vi "Set XY Scale Properties on Variant.vi"(8 "error in (no error)":errorcluster, 10 "Scale Properties":T1 {"X.Format" items=["Decimal", "Scientific", "Engineering", "Binary", "Octal", "Hexadecimal", "Relative Time", "Time and Date", "SI", "Automatic"]; "Y.Precision:" items=["0", "1", "2", "3", "4", "5", "6", "7"]; "Y.Format" items=["Decimal", "Scientific", "Engineering", "Binary", "Octal", "Hexadecimal", "Relative Time", "Time and Date", "SI", "Automatic"]; "X.Precision" items=["0", "1", "2", "3", "4", "5", "6", "7"]}, 11 "variant in":variant) -> (0 "error out":errorcluster, 3 "variant out":variant)   [LabVIEW 2020, in "Workspace MultiY Graph.lvlib"]
uses:
  Workspace MultiY Graph.lvlib
  XY Scale Properties.ctl
  XY Scale Precision.ctl
  XY Scale Format.ctl
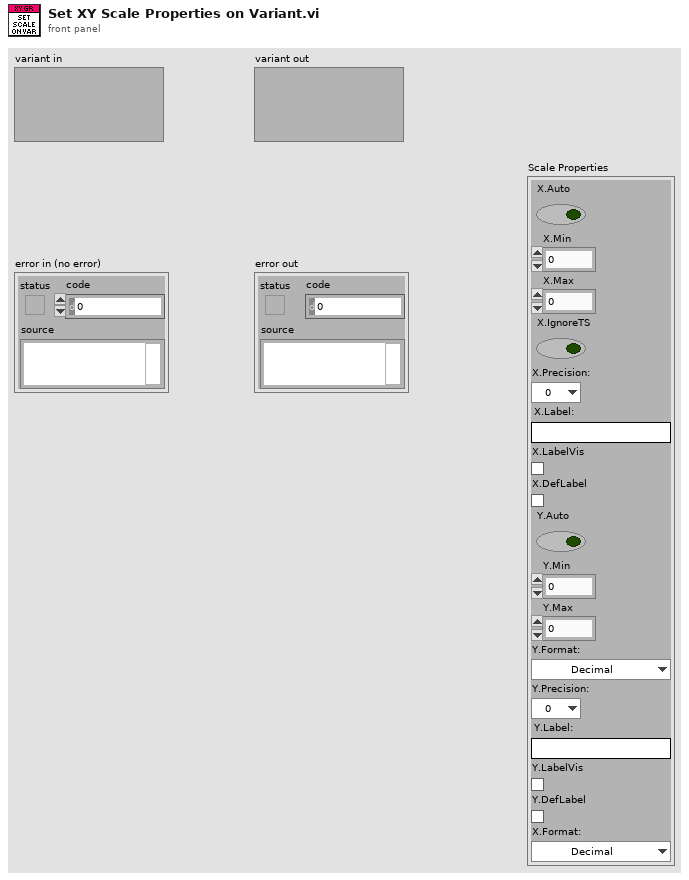
[diagram p1: front panel]
types:
  T1 = typedef "Workspace MultiY Graph.lvlib/XY Scale Properties.ctl" = cluster{"X.Auto":bool, "X.Min":dbl, "X.Max":dbl, "X.IgnoreTS":bool, "X.Precision":T2, "X.Label:":string, "X.LabelVis":bool, "X.DefLabel":bool, "Y.Auto":bool, "Y.Min":dbl, "Y.Max":dbl, "Y.Format":T3, "Y.Precision:":T2, "Y.Label:":string, "Y.LabelVis":bool, "Y.DefLabel":bool, "X.Format":T3}
  T2 = typedef "Workspace MultiY Graph.lvlib/XY Scale Precision.ctl" = u8
  T3 = typedef "Workspace MultiY Graph.lvlib/XY Scale Format.ctl" = u8
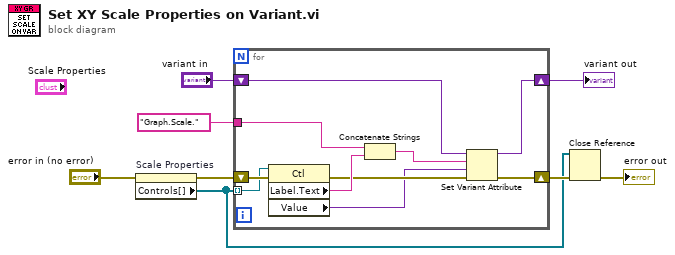
[diagram p0: block diagram]
diagram:
  n1 = property on="Scale Properties" class="Clust (strict)"(error in="error in (no error)") -> (error out=w8:errorcluster, "Controls[]"=w4:refnum<vi>[])  [unwired: 1 in, 1 out]
  n2 = for {
    tunnel: w4 -> [w17] mode=indexing
    tunnel: "Graph.Scale." ("name") -> [w15]
    shift-right: [w16] -> w5
    shift-left: w8 -> [w18]
    shift-right: [w13] -> w6
    shift-left: "variant in" -> [w14]
    n3 = property on="Property Node" class="Ctl"(reference=w17, error in=w18) -> (error out=w11:errorcluster, "Label.Text"=w12:string, "Value"=w9:variant)  [unwired: 1 out]
    n4 = Concatenate Strings(w15, w12) -> (w10:string)
    n5 = Set Variant Attribute(Variant=w14, name=w10, value=w9, error in=w11) -> (Variant out=w13:variant, error out=w16:errorcluster)  [unwired: 1 out]
  }
  "variant out" <- w6
  n6 = Close Reference(reference=w4, error in (no error)=w5) -> (error out=→"error out":errorcluster)
